vi "Write move index.vi"(8 "error in (no error)":errorcluster, 10 "move index":i32, 11 "MotorSim in":refnum<class "MotorSim.lvclass">) -> (0 "error out":errorcluster, 3 "MotorSim out":refnum<class "MotorSim.lvclass">)   [LabVIEW 2018, in "MotorSim.lvclass"]
uses:
  MotorSim.lvclass
  MotorSim.lvclass/MotorSim.ctl
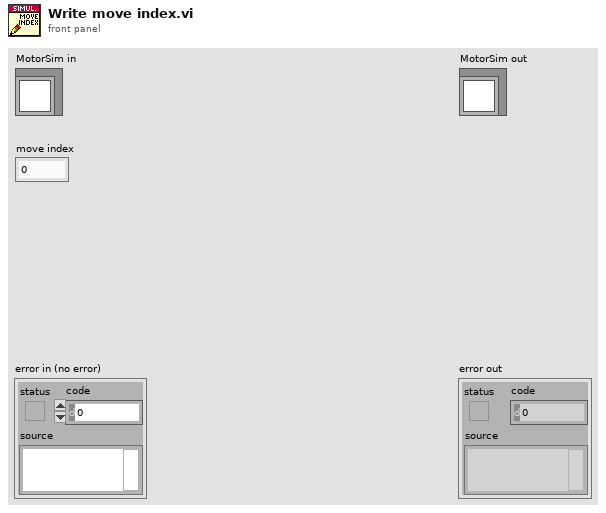
[diagram p1: front panel]
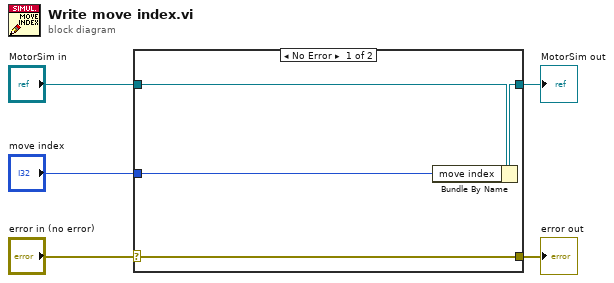
[diagram p0: block diagram]
diagram:
  n1 = case shown="No Error" "error in (no error)" {
    selector: "error in (no error)" -> [w9 w10]
    tunnel: [w9 w10] -> w4
    tunnel: [w7 w11] -> w2
    tunnel: "MotorSim in" -> [w8 w11]
    tunnel: "move index" -> [w6 _]
    frame No Error {
      n2 = Bundle By Name(cluster=w8, "move index"=w6) -> (w7:refnum<class "MotorSim.lvclass">)
    }
    frame Error {
    }
  }
  "error out" <- w4
  "MotorSim out" <- w2
